vi "json_to_dictionary.vi"(8 "error in (no error)":errorcluster, 11 "json_path":path) -> (0 "error out":errorcluster, 3 "units []":T1[](array[typedef]))   [LabVIEW 2015, in "lv-unit-conversion.lvlib"]
uses:
  lv-unit-conversion.lvlib
  public/_controls/unit.ctl
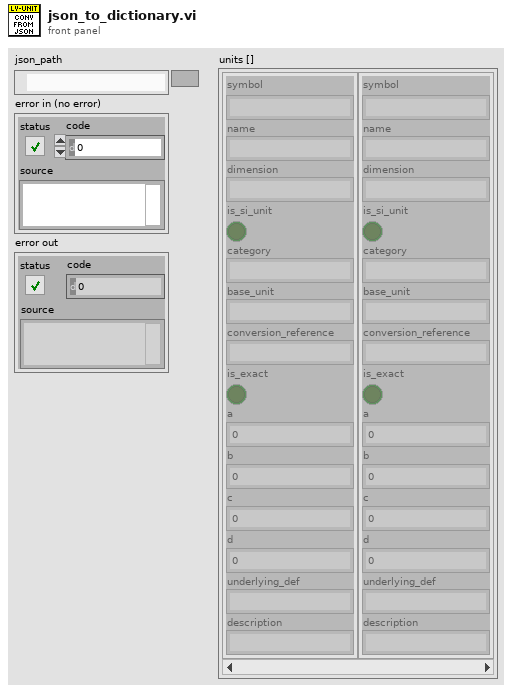
[diagram p1: front panel]
types:
  T1 = typedef "lv-unit-conversion.lvlib/unit.ctl" = cluster{"symbol":string, "name":string, "dimension":string, "is_si_unit":bool, "category":string, "base_unit":string, "conversion_reference":string, "is_exact":bool, "a":dbl, "b":dbl, "c":dbl, "d":dbl, "underlying_def":string, "description":string}
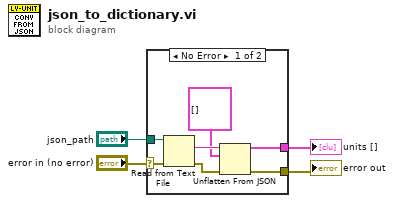
[diagram p0: block diagram]
diagram:
  n1 = case shown="No Error" "error in (no error)" {
    selector: "error in (no error)" -> [w10 w12]
    tunnel: [w6 w12] -> w3
    tunnel: "json_path" -> [w11 _]
    tunnel: [w5 _] -> w1
    frame No Error {
      n2 = Read from Text File(file (use dialog)=w11, error in=w10) -> (text=w9:string, error out=w7:errorcluster)  [unwired: 2 in, 2 out]
      n3 = Unflatten From JSON(JSON string=w9, type and defaults=T1[] [] ("data_set"), error in (no error)=w7) -> (value=w5:T1[], error out=w6:errorcluster)  [unwired: 4 in]
    }
    frame Error {
    }
  }
  "error out" <- w3
  "units []" <- w1
